vi "SubtractPlots.vi"(10 "Set 2":cluster{"x0":dbl, "df":dbl, dbl[]}, 11 "Set 1":cluster{"x0":dbl, "df":dbl, dbl[]}) -> (3 "Difference":cluster{"x0":dbl, "df":dbl, dbl[]})   [LabVIEW 2022 SP3]
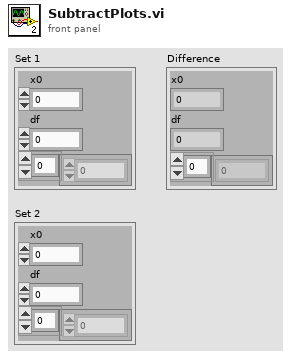
[diagram p1: front panel]
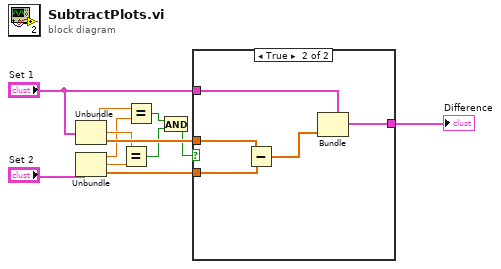
[diagram p0: block diagram]
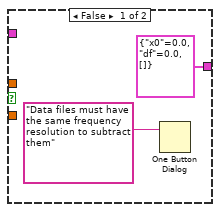
[diagram p2: hidden frame]
diagram:
  n1 = Unbundle("Set 1") -> ("x0"=w5:dbl, "df"=w6:dbl, w9:dbl[])
  n2 = Unbundle("Set 2") -> ("x0"=w4:dbl, "df"=w7:dbl, w8:dbl[])
  n3 = Equal?(x=w6, y=w7) -> (x = y?=w2:bool)
  n4 = Equal?(x=w5, y=w4) -> (x = y?=w3:bool)
  n5 = And(x=w3, y=w2) -> (x .and. y?=w1:bool)
  n6 = case shown="True" w1 {
    tunnel: [cluster{"x0":dbl, "df":dbl, dbl[]} {"x0"=0.0, "df"=0.0, []} ("Set 1") w19] -> w11
    tunnel: "Set 1" -> [_ w17]
    tunnel: w9 -> [_ w16]
    tunnel: w8 -> [_ w15]
    frame False {
      n7 = One Button Dialog(message="Data files must have the same frequency resolution to subtract them") -> ()  [unwired: 1 in, 1 out]
    }
    frame True {
      n8 = Subtract(x=w16, y=w15) -> (x-y=w18:dbl[])
      n9 = Bundle(cluster=w17, w18) -> (w19:cluster{"x0":dbl, "df":dbl, dbl[]})  [unwired: 2 in]
    }
  }
  "Difference" <- w11
